vi "COMI US Get Buf Ptr.vi"(11 "hDevice":u32) -> (2 "function return":i16, 3 "hDevice out":u32)   [LabVIEW 2017, in "Comidll.lvlib"]
doc: "short (COMI_US_GetBufPtr) (HANDLE hDevice);"
uses:
  <userlib>/Comidll/Comidll.lvlib
  <userlib>/Comidll/Comidll.dll
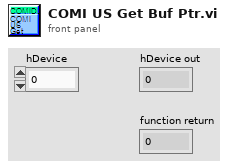
[diagram p1: front panel]
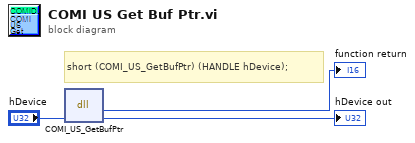
[diagram p0: block diagram]
diagram:
  # "short\t(COMI_US_GetBufPtr) (HANDLE hDevice);"
  n1 = dll-call lib="C:/Program Files/National Instruments/LabVIEW 2017/user.lib/Comidll/Comidll.*" fn="COMI_US_GetBufPtr"("hDevice"="hDevice") -> (→"function return":i16, "hDevice"=→"hDevice out":u32)  [unwired: 3 in, 2 out]
